vi "HR_Calculate_Percentage.vi"(7 "error in (no error)":errorcluster, 10 "HR Data Structure in":T3) -> (0 "error out":errorcluster, 2 "reversed array":dbl[](array[numeric]), 3 "ShowCluster":T2)   [LabVIEW 2021]
doc: "This Vi calculetes how much training time runner spends in each zone and writes it to clutes and double array"
uses:
  Controls/HR Data Structure.ctl
  Controls/Runner's Data.ctl
  Controls/Raw Data.ctl
  e6a1e60f-9a01-4349-afc9-f9c02ba13944.vi
  <vilib>/Comparison/Less/Less Functor/Less Functor.lvclass
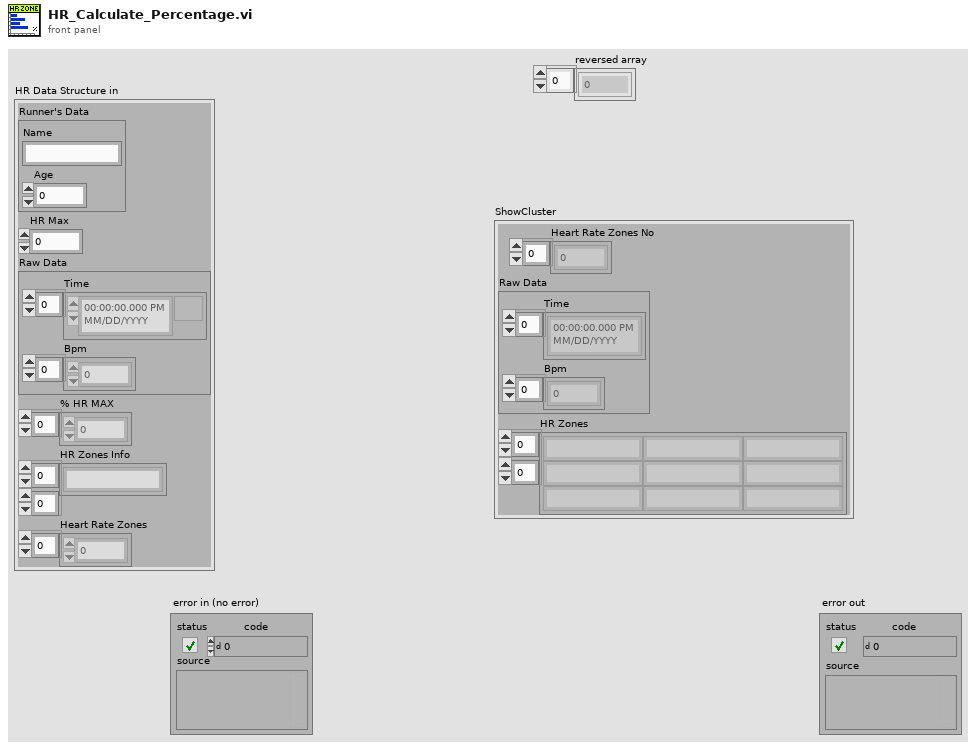
[diagram p1: front panel]
types:
  T1 = typedef "Raw Data.ctl" = cluster{"Time":timestamp[], "Bpm":i32[]}
  T2 = cluster{"Heart Rate Zones No":dbl[], "Raw Data":T1, "HR Zones":string[][]}
  T3 = typedef "HR Data Structure.ctl" = cluster{"Runner's Data":T4, "HR Max":i32, "Raw Data":T1, "% HR MAX ":dbl[], "HR Zones Info":string[][], "Heart Rate Zones":dbl[]}
  T4 = typedef "Runner's Data.ctl" = cluster{"Name":string, "Age":i32}
  T5 = cluster{i32[], "Raw Data":T1, "HR Zones Info":string[][]}
  T6 = cluster{"Heart Rate Zones":dbl[], "Raw Data":T1, "HR Zones Info":string[][]}
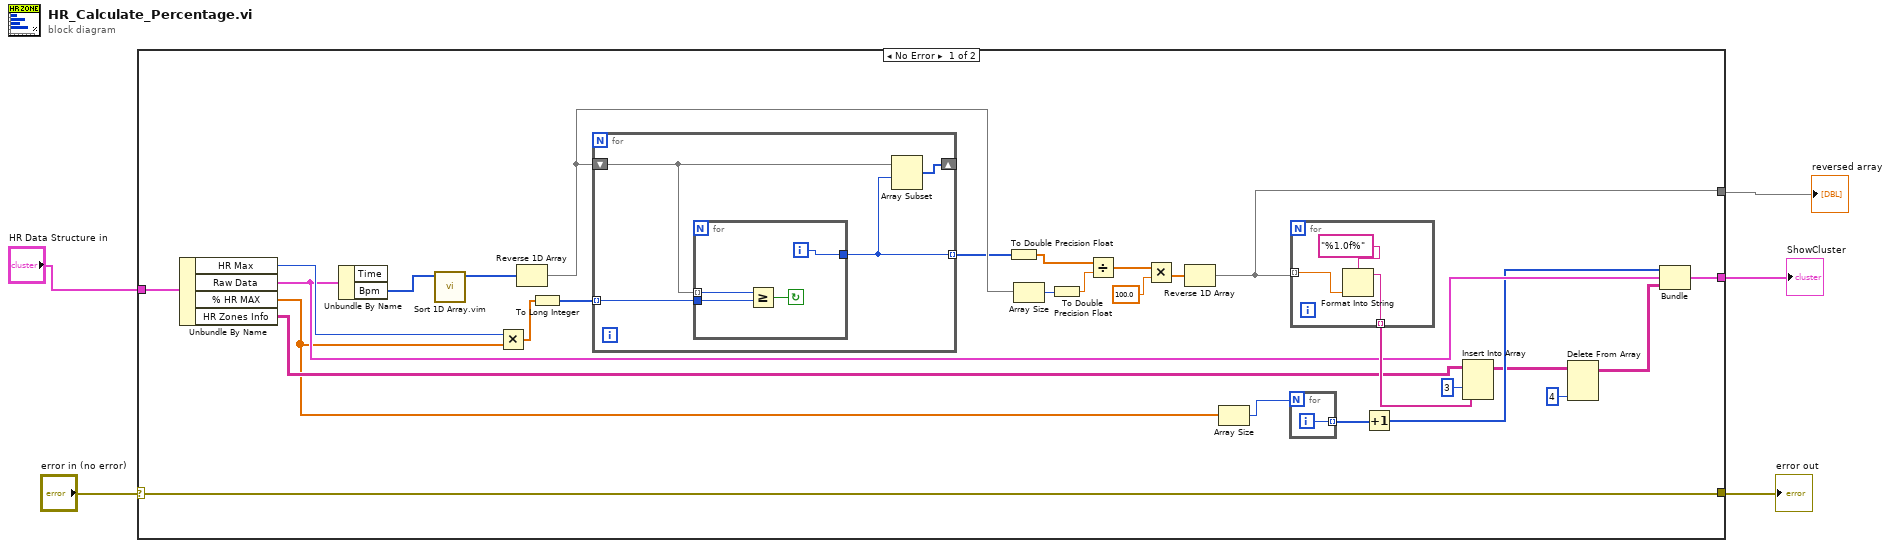
[diagram p0: block diagram]
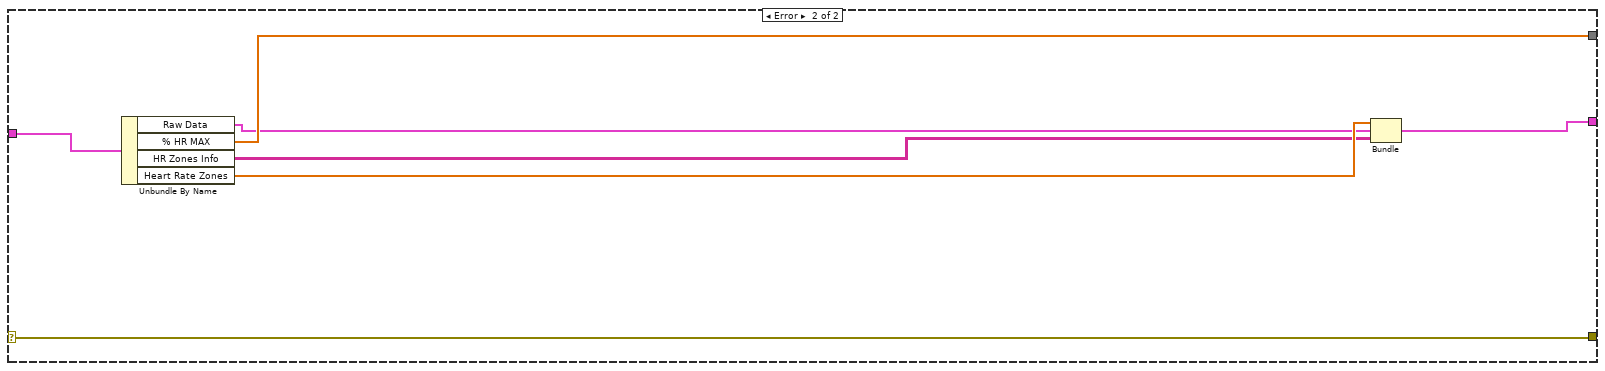
[diagram p2: hidden frame]
diagram:
  n1 = case shown="No Error" "error in (no error)" {
    selector: "error in (no error)" -> [w20 w52]
    tunnel: "HR Data Structure in" -> [w9 w51]
    tunnel: [w20 w52] -> w3
    tunnel: [w17 w50] -> w2
    tunnel: [w10 w49] -> w1
    frame No Error {
      n2 = Unbundle By Name(w9) -> ("HR Max"=w32:i32, "Raw Data"=w16:T1, "% HR MAX"=w14:dbl[], "HR Zones Info"=w18:string[][])
      n3 = Unbundle By Name(w16) -> ("Bpm"=w31:i32[])  [unwired: 1 out]
      n4 = call "Sort 1D Array.vim"("unsorted array"=w31) -> ("sorted array"=w21:i32[])  [unwired: 10 in]
      n5 = Multiply(x=w32, y=w14) -> (x*y=w33:dbl[])
      n6 = Reverse 1D Array(array=w21) -> (reversed array=w23:i32[])
      n7 = To Long Integer(number=w33) -> (32bit integer=w30:i32[])
      n8 = for {
        shift-right: [w40] -> _
        shift-left: w23 -> [w41]
        tunnel: [w39] -> w22 mode=indexing
        tunnel: w30 -> [w38] mode=indexing
        n9 = for {
          tunnel: w41 -> [w42] mode=indexing
          tunnel: [w45] -> w39
          tunnel: w38 -> [w43]
          i -> [w45]
          stop <- w44 continue-if-true
          n10 = Greater Or Equal?(x=w42, y=w43) -> (x >= y?=w44:bool)
        }
        n11 = Array Subset(array=w41, index=w39) -> (w40:i32[])  [unwired: 1 in]
      }
      n12 = To Double Precision Float(number=w22) -> (double precision float=w26:dbl[])
      n13 = Array Size(array=w23) -> (size(s)=w24:i32)
      n14 = To Double Precision Float(number=w24) -> (double precision float=w25:dbl)
      n15 = Divide(x=w26, y=w25) -> (x/y=w28:dbl[])
      n16 = Multiply(x=w28, y=100.0) -> (x*y=w29:dbl[])
      n17 = Reverse 1D Array(array=w29) -> (reversed array=w17:dbl[])
      n18 = Array Size(array=w14) -> (size(s)=w13:i32)
      n19 = for {
        N: w13 -> [_]
        tunnel: [w34] -> w12 mode=indexing
        i -> [w34]
      }
      n20 = for {
        tunnel: w17 -> [w36] mode=indexing
        tunnel: [w35] -> w19 mode=indexing
        n21 = Format Into String(format string="%1.0f%", w36) -> (resulting string=w35:string)  [unwired: 2 in, 1 out]
      }
      n22 = Increment(x=w12) -> (x+1=w11:i32[])
      n23 = Insert Into Array(array=w18, index (col)=3 ("disabled index (col)"), new element=w19) -> (w7:string[][])  [unwired: 1 in]
      n24 = Delete From Array(array=w7, index (col)=4 ("disabled index (col)")) -> (array with subset deleted=w8:string[][])  [unwired: 2 in, 1 out]
      n25 = Bundle(w11, "Raw Data"=w16, "HR Zones Info"=w8) -> (w10:T5)  [unwired: 1 in]
    }
    frame Error {
      n26 = Unbundle By Name(w51) -> ("Raw Data"=w47:T1, "% HR MAX"=w50:dbl[], "HR Zones Info"=w46:string[][], "Heart Rate Zones"=w48:dbl[])
      n27 = Bundle("Heart Rate Zones"=w48, "Raw Data"=w47, "HR Zones Info"=w46) -> (w49:T6)  [unwired: 1 in]
    }
  }
  "error out" <- w3
  "reversed array" <- w2
  "ShowCluster" <- w1
